vi "c ctre phoenixpro serialize pgn no malloc.vi"(6 "max_len":u32, 7 "str":string, 8 "error in (no error)":errorcluster, 9 "framePeriodMs":u16, 10 "frame_index":u16, 11 "spn":i32) -> (0 "error out":errorcluster, 3 "function return":i32, 5 "str out":string)   [LabVIEW 2020, in "CTRE_PhoenixTools.lvlib"]
doc: "CTREXPORT int c_ctre_phoenixpro_serialize_pgn_no_malloc(int spn, uint16_t frame_index, uint16_t framePeriodMs, char *str, uint32_t max_len);"
uses:
  <userlib>/CTRE_PhoenixTools/CTRE_PhoenixTools.lvlib
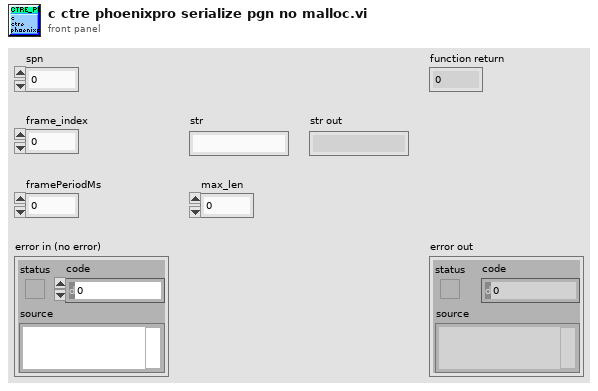
[diagram p1: front panel]
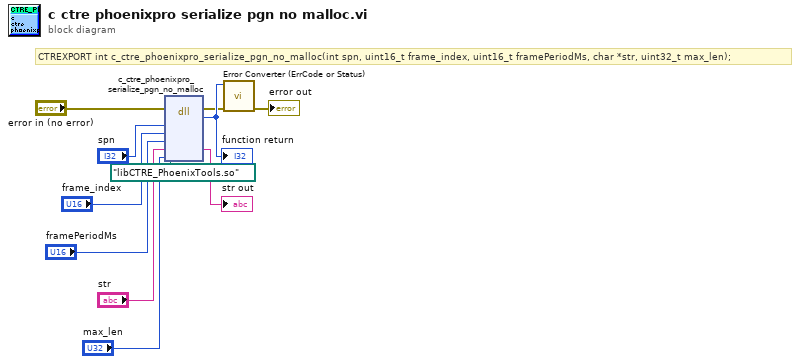
[diagram p0: block diagram]
diagram:
  # "CTREXPORT int c_ctre_phoenixpro_serialize_pgn_no_malloc(int spn, uint16_t frame_index, uint16_t framePeriodMs, char *str, uint32_t max_len);"
  n1 = dll-call lib="?" fn="c_ctre_phoenixpro_serialize_pgn_no_malloc"(path in=path "libCTRE_PhoenixTools.so", error in="error in (no error)", "spn"="spn", "frame_index"="frame_index", "framePeriodMs"="framePeriodMs", "str"="str", "max_len"="max_len") -> (error out=w3:errorcluster, w11:i32, "str"=→"str out":string)  [unwired: 5 in, 1 out]
  "function return" <- w11
  n2 = call <userlib>:"Error Converter (ErrCode or Status).vi"("error in (no error)"=w3, "error code"=w11) -> ("error out"=→"error out":errorcluster)  [unwired: 9 in]
